vi "Empty.vi"() -> ()   [LabVIEW 2017, in "Assertions.Tests.lvlib" / "Assert Not Count.lvlib"]
uses:
  Assert Not Count.lvlib
  src/Transparent Assertions/Assertions/Assertions.lvlib
panel:
  out "error out":errorcluster
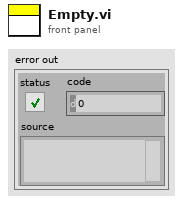
[diagram p1: front panel]
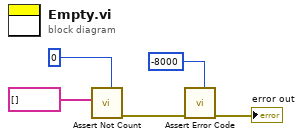
[diagram p0: block diagram]
diagram:
  n1 = call "Assert Not Count.vi"("Expected"=0, "Haystack"=string[] []) -> ("error out"=w3:errorcluster)  [unwired: 9 in]
  n2 = call "Assert Error Code.vi"("Expected"=-8000, "error in (no error)"=w3) -> ("error out"=→"error out":errorcluster)  [unwired: 9 in]
